vi "Average_complete.vi"(0 "VISA resource name":refnum<visa-resource-name>, 1 "error in (no error)":errorcluster) -> (2 "VISA resource name out":refnum<visa-resource-name>, 3 "Average Complete":bool, 4 "error out":errorcluster)   [LabVIEW 2020]
uses:
  <instrlib>/Keysight PNA Series/Keysight PNA Series.lvlib
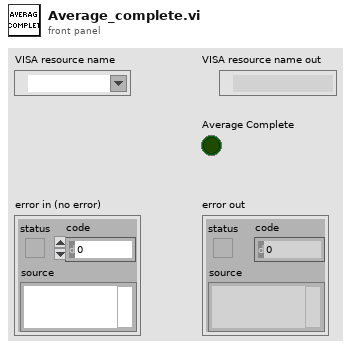
[diagram p1: front panel]
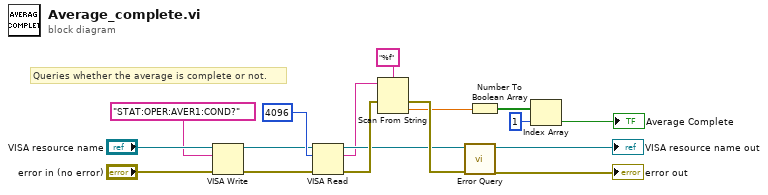
[diagram p0: block diagram]
diagram:
  # "Queries whether the average is complete or not."
  n1 = VISA Write(VISA resource name="VISA resource name", write buffer="STAT:OPER:AVER1:COND?", error in (no error)="error in (no error)") -> (VISA resource name out=w14:refnum<visa-resource-name>, error out=w13:errorcluster)  [unwired: 1 out]
  n2 = VISA Read(VISA resource name=w14, byte count=4096, error in (no error)=w13) -> (VISA resource name out=w7:refnum<visa-resource-name>, read buffer=w6:string, error out=w9:errorcluster)  [unwired: 1 out]
  n3 = Scan From String(format string="%f", input string=w6, error in=w9) -> (error out=w8:errorcluster, output 1=w4:dbl)  [unwired: 2 in, 2 out]
  n4 = call <instrlib>:"Error Query.vi"("error in (no error)"=w8, "VISA resource name"=w7) -> ("error out"=→"error out":errorcluster, "VISA resource name out"=→"VISA resource name out":refnum<visa-resource-name>)  [unwired: 6 in, 2 out]
  n5 = Number To Boolean Array(number=w4) -> (Boolean array=w3:bool[])
  n6 = Index Array(array=w3, index=1) -> (element=→"Average Complete":bool)
